vi "Set DDS Duty Cycle.vi"(10 "cycle":i32, 11 "channel_index":u8) -> ()   [LabVIEW 2021, in "vmmso.lvlib"]
doc: "DLL_API void WINAPI SetDDSDutyCycle(unsigned char channel_index, int cycle);"
uses:
  vmmso.lvlib
  vmmso.dll
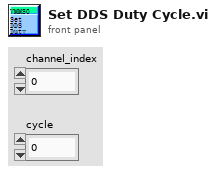
[diagram p1: front panel]
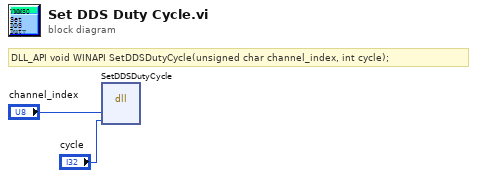
[diagram p0: block diagram]
diagram:
  # "DLL_API void WINAPI SetDDSDutyCycle(unsigned char channel_index, int cycle);"
  n1 = dll-call lib="D:/labviewdemo/LabviewDemo 21/vmmso/vmmso.*" fn="SetDDSDutyCycle"("channel_index"="channel_index", "cycle"="cycle") -> ()  [unwired: 6 in, 2 out]
